vi "Configure.vi"(8 "error in (no error)":errorcluster) -> (0 "error out":errorcluster, 1 "valid config":bool, 3 "config":T1)   [LabVIEW 2017, in "OpState.lvlib"]
uses:
  <vilib>/addons/InsightCM/Devices/Shared/Common/OpState/OpState.lvlib
  <vilib>/addons/InsightCM/Devices/Shared/Common/OpState/controls/config.ctl
  <vilib>/addons/InsightCM/Utilities/GlobalConfiguration/GlobalConfiguration.lvlib
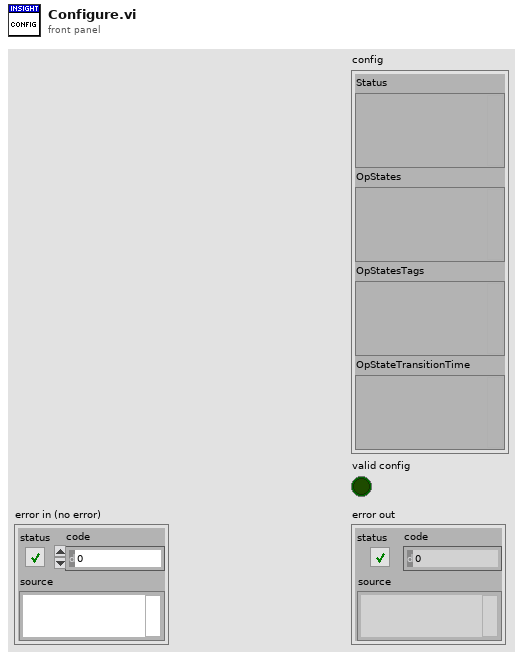
[diagram p1: front panel]
types:
  T1 = typedef "OpState.lvlib/config.ctl" = cluster{"Status":variant, "OpStates":variant, "OpStatesTags":variant, "OpStateTransitionTime":variant}
  T2 = typedef "R2_Device.ctl" = cluster{"Id":string, "Name":string, "DeviceType":string, "HardwareName":string, "IpAddress":string, "HardwareInfo":T3[], "ApplicationType":string, "ApplicationVersion":string, "EquipmentIds":string[], "ConfigurationVersion":string, "State":T4, "Properties":T3[], "DataGroups":T5[], "BurstModeTrigger":T9}
  T3 = typedef "KeyValuePair.ctl" = cluster{"Key":string, "Value":string}
  T4 = typedef "DeviceState.ctl" = cluster{"Disabled":bool}
  T5 = typedef "R2_DataGroup.ctl" = cluster{"Name":string, "OperatingStates":T6[], "Properties":T3[], "EquipmentIds":string[], "AssetNodeId":string}
  T6 = typedef "OperatingState.ctl" = cluster{"Name":string, "Properties":T3[], "Triggers":T7[]}
  T7 = typedef "Trigger.ctl" = cluster{"Type":string, "Expression":string, "Conditions":T8[]}
  T8 = typedef "Condition.ctl" = cluster{"Source":string, "Type":string, "Operator":string, "CompareTo":string, "DwellSeconds":dbl}
  T9 = typedef "BurstModeTrigger.ctl" = cluster{"Trigger":T7, "SampleRate":string, "AcquisitionLength":string}
  T10 = typedef "ConfigListItem.ctl" = cluster{"Id":string, "Name":string, "ReadOnly":bool, "Weight":i32}
  T11 = typedef "MetricDefinitionInstance.ctl" = cluster{"Id":string, "MetricType":string, "Name":string, "Properties":T3[], "HighRate":bool}
  T12 = typedef "SectionKeyValues.ctl" = cluster{"Section":string, "KeyValues":T3[]}
  T13 = typedef "AssetNode.ctl" = cluster{"Id":string, "Type":string, "Name":string, "ParentIds":string[], "State":T14, "MeasType":string, "Properties":T3[], "OperatingStates":T6[], "Metrics":T15[], "TrendAlarmRules":T16[], "References":T19[]}
  T14 = typedef "AssetState.ctl" = cluster{"Disabled":bool}
  T15 = typedef "Metric.ctl" = cluster{"Id":string, "Name":string, "Unit":string, "Properties":T3[], "MetricDefinitionInstanceId":string}
  T16 = typedef "TrendAlarmRule.ctl" = cluster{"Id":string, "AssetNodeId":string, "TrendId":string, "Disabled":bool, "OperatingState":string, "Operator":string, "Hysteresis":dbl, "OnDelaySeconds":dbl, "OffDelaySeconds":dbl, "Levels":T17[], "Properties":T3[]}
  T17 = typedef "TrendAlarmLevel.ctl" = cluster{"Severity":i32, "CompareTo":dbl, "Actions":T18[]}
  T18 = typedef "AlarmAction.ctl" = cluster{"Type":string, "Props":T3[]}
  T19 = typedef "AssetNodeReference.ctl" = cluster{"NodeId":string, "Name":string}
  T20 = typedef "R2_Channel.ctl" = cluster{"Id":string, "DeviceId":string, "Name":string, "ChannelType":string, "HardwareKey":string, "HardwareChannel":string, "DataGroup":string, "Keywords":string[], "EquipmentIds":string[], "Properties":T3[], "Metrics":T15[], "AssetNodeId":string, "MeasType":string, "AssetName":string}
  T21 = typedef "Tag.ctl" = cluster{"Id":string, "Path":string, "Name":string, "Datatype":string, "Props":T3[], "Keywords":string[]}
  T22 = typedef "OpState.lvlib/TriggerOperatingState.ctl" = cluster{"Id":string, "Name":string, "Properties":T3[], "EnterExpression":string, "EnterConditions":T23[], "ExitExpression":string, "ExitConditions":T23[]}
  T23 = typedef "Trigger.lvlib/TriggerCondition.ctl" = cluster{"Condition":T8, "LatchValue":string, "LatchTime":timestamp}
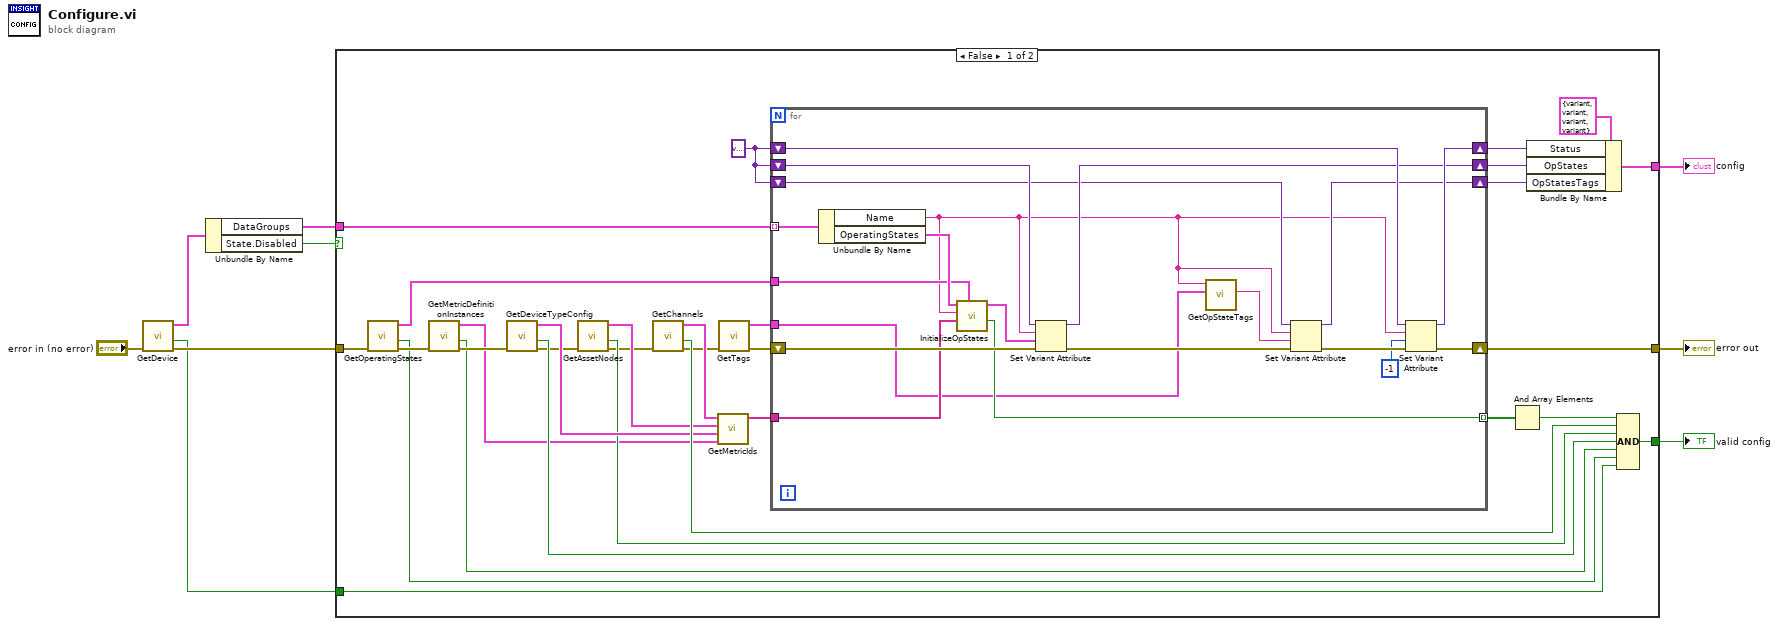
[diagram p0: block diagram]
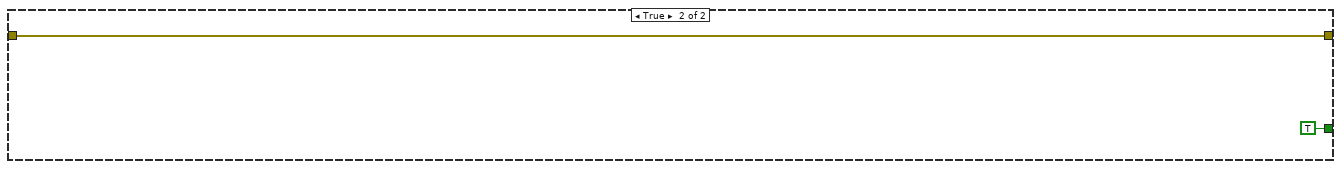
[diagram p2: hidden frame]
diagram:
  n1 = call <vilib>:"GetDevice.vi"("error in (no error)"="error in (no error)") -> ("error out"=w3:errorcluster, "found"=w2:bool, "device configuration"=w8:T2)  [unwired: 8 in]
  n2 = Unbundle By Name(w8) -> ("DataGroups"=w7:T5[], "State.Disabled"=w1:bool)
  n3 = case shown="False" w1 {
    tunnel: w7 -> [w40 _]
    tunnel: [w39 w62] -> w6
    tunnel: [w38 _] -> w5
    tunnel: [w33 TRUE] -> w4
    tunnel: w3 -> [w21 w62]
    tunnel: w2 -> [w19 _]
    frame False {
      w12 = variant ("Status")
      n4 = call <vilib>:"GetOperatingStates.vi"("error in (no error)"=w21) -> ("error out"=w20:errorcluster, "found"=w18:bool, "OperatingStates"=w17:T10[])  [unwired: 8 in]
      n5 = call <vilib>:"GetMetricDefinitionInstances.vi"("error in (no error)"=w20) -> ("error out"=w24:errorcluster, "found"=w23:bool, "metrics"=w22:T11[])  [unwired: 8 in]
      n6 = call <vilib>:"GetDeviceTypeConfig.vi"("error in (no error)"=w24) -> ("error out"=w25:errorcluster, "found"=w29:bool, "key values"=w30:T12[])  [unwired: 8 in]
      n7 = call <vilib>:"GetAssetNodes.vi"("error in (no error)"=w25) -> ("error out"=w26:errorcluster, "found"=w27:bool, "AssetNodes"=w28:T13[])  [unwired: 8 in]
      n8 = call <vilib>:"GetChannels.vi"("error in (no error)"=w26) -> ("error out"=w31:errorcluster, "found"=w32:bool, "channels"=w35:T20[])  [unwired: 8 in]
      n9 = call <vilib>:"GetMetricIds.vi"("metrics"=w22, "device type config"=w30, "AssetNodes"=w28, "channels"=w35) -> ("metric ids"=w34:string[])  [unwired: 7 in]
      n10 = call <vilib>:"GetTags.vi"("error in (no error)"=w31) -> ("error out"=w37:errorcluster, "tags"=w36:T21[])  [unwired: 8 in, 1 out]
      n11 = for {
        tunnel: w40 -> [w60] mode=indexing
        shift-right: [w57] -> w16
        shift-left: w12 -> [w58]
        shift-right: [w55] -> w15
        shift-left: w12 -> [w59]
        shift-right: [w48] -> w39
        shift-left: w37 -> [w49]
        shift-right: [w51] -> w13
        shift-left: w12 -> [w52]
        tunnel: w36 -> [w43]
        tunnel: w34 -> [w46]
        tunnel: [w45] -> w11 mode=indexing
        tunnel: w17 -> [w44]
        n12 = Unbundle By Name(w60) -> ("Name"=w42:string, "OperatingStates"=w50:T6[])
        n13 = call <vilib>:"InitializeOpStates.vi"("op state defs"=w44, "metric ids"=w46, "data group name"=w42, "operating states in"=w50) -> ("valid config"=w45:bool, "sorted operating states"=w56:T22[])  [unwired: 6 in]
        n14 = Set Variant Attribute(Variant=w59, name=w42, value=w56, error in=w49) -> (Variant out=w55:variant, error out=w54:errorcluster)  [unwired: 1 out]
        n15 = call <vilib>:"GetOpStateTags.vi"("tags"=w43, "data group"=w42) -> ("op state tag id"=w41:string)  [unwired: 9 in]
        n16 = Set Variant Attribute(Variant=w52, name=w42, value=w41, error in=w54) -> (Variant out=w51:variant, error out=w53:errorcluster)  [unwired: 1 out]
        n17 = Set Variant Attribute(Variant=w58, name=w42, value=-1 ("CurrentOpState"), error in=w53) -> (Variant out=w57:variant, error out=w48:errorcluster)  [unwired: 1 out]
      }
      n18 = And Array Elements(Boolean array=w11) -> (logical AND=w10:bool)
      n19 = Bundle By Name(cluster=T1 {"Status"=variant, "OpStates"=variant, "OpStatesTags"=variant, "OpStateTransitionTime"=variant} ("config"), "Status"=w16, "OpStates"=w15, "OpStatesTags"=w13) -> (w38:T1)
      n20 = Compound Arithmetic op=AND(w10, w32, w27, w29, w23, w18, w19) -> (w33:bool)
    }
    frame True {
    }
  }
  "error out" <- w6
  "config" <- w5
  "valid config" <- w4
